vi "Format OpCode.vi"(4 "Format":T1) -> (7 "OpCode":T2)   [LabVIEW 2020, in "HTTP Server.lvlib" / "WebSocket Client.lvclass"]
uses:
  WebSocket Client.lvclass
  WebSocket Client.lvclass/WebSocket Client.ctl
  OpCode.ctl
  WebSocket Format.ctl
  HTTP Server.lvlib
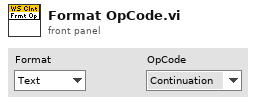
[diagram p1: front panel]
types:
  T1 = typedef "HTTP Server.lvlib/WebSocket Format.ctl" = enum16{"Text", "Binary"}
  T2 = typedef "HTTP Server.lvlib/WebSocket Client.lvclass/OpCode.ctl" = enum8{"Continuation", "Text", "Binary", "Reserved3", "Reserved4", "Reserved5", "Reserved6", "Reserved7", "Close", "Ping", "Pong", "ReservedB", "ReservedC", "ReservedD", "ReservedE", "ReservedF"}
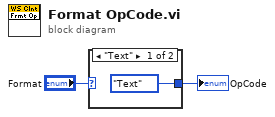
[diagram p0: block diagram]
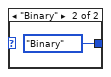
[diagram p2: hidden frame]
diagram:
  n1 = case shown="\"Text\"" "Format" {
    tunnel: [OpCode."Text" ("OpCode") OpCode."Binary" ("OpCode")] -> w1
    frame "Text" {
    }
    frame "Binary" {
    }
  }
  "OpCode" <- w1
